vi "Get Type.vi"(11 "Boolean 1D in":refnum<class "Assertion 1D.lvclass">) -> (3 "Type":string)   [LabVIEW 2017, in "Assertion 1D.lvclass"]
uses:
  <vilib>/gpm_packages/@cs/data-type-serializer/source/Assertion 1D/Assertion 1D.lvclass
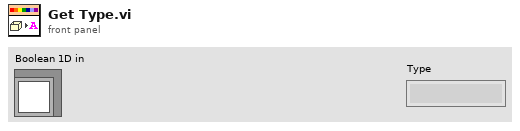
[diagram p1: front panel]
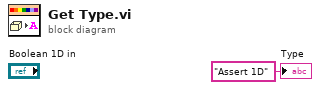
[diagram p0: block diagram]
diagram:
  "Type" <- "Assert 1D" ("Type")
